vi "prepare16.vi"(6 "pzTail":u32, 7 "ppStmt":dbl, 8 "error in (no error)":errorcluster, 9 "nByte":i32, 10 "zSql":u32, 11 "db":dbl) -> (0 "error out":errorcluster, 2 "function return":i32, 3 "db out":dbl, 5 "ppStmt out":dbl)   [LabVIEW 2020, in "sqlite3.lvlib"]
uses:
  sqlite3.lvlib
  errstr.vi
  bin/sqlite3_64.dll
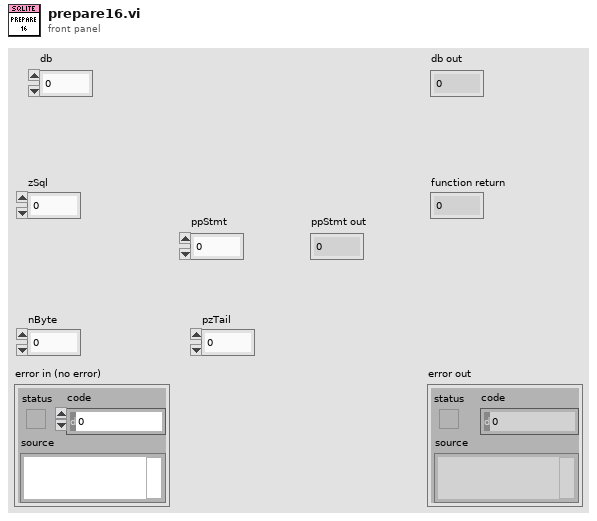
[diagram p1: front panel]
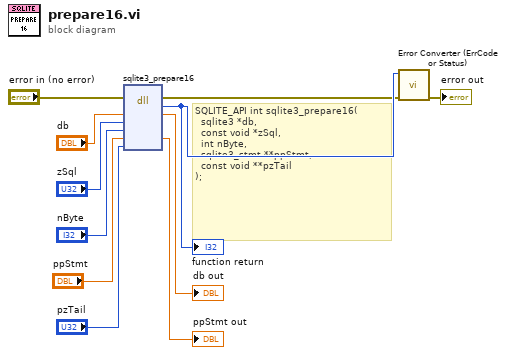
[diagram p0: block diagram]
diagram:
  # "SQLITE_API int sqlite3_prepare16(\n  sqlite3 *db,            \n  const void *zSql,       \n  int nByte,              \n  sqlite3_stmt **ppStmt,  \n  const void **pzTail     \n);"
  n1 = dll-call lib="C:/Users/Fred.Guo/Desktop/Database-configuration/externals/sqlite3/Source/bin/sqlite3_*.*" fn="sqlite3_prepare16"(error in="error in (no error)", "db"="db", "zSql"="zSql", "nByte"="nByte", "ppStmt"="ppStmt", "pzTail"="pzTail") -> (error out=w2:errorcluster, w11:i32, "db"=→"db out":dbl, "ppStmt"=→"ppStmt out":dbl)  [unwired: 5 in, 1 out]
  "function return" <- w11
  n2 = call "Error Converter (ErrCode or Status).vi"("error in (no error)"=w2, "error code"=w11) -> ("error out"=→"error out":errorcluster)  [unwired: 9 in]
